vi "PV ActiveLine - Sensor On-Off (TPG361).vi"(7 "W/R":bool, 8 "Fehler (Eingang)":errorcluster, 10 "Sensor 1 Set":u8(ring) items=["No status change", "Turn gauge off", "Turn gauge on"], 11 "Referenz in":refnum<visa-resource-name>) -> (0 "Cluster (Ausgang)":errorcluster, 2 "Sensor 1 Set":u8(ring) items=["Gauge cannot be turned on/off", "Gauge turned off", "Gauge turned on"], 3 "Referenz out":refnum<visa-resource-name>)   [LabVIEW 2013, in "PV ActiveLine.lvlib"]
doc: "SEN - Turning a Gauge on/off\n\nTransmit: SEN [,a]\n\nGauge 1,\na =\n0 –> No status change\n1 –> Turn gauge off\n2 –> Turn gauge on"
uses:
  <instrlib>/PV ActiveLine/PV ActiveLine.lvlib
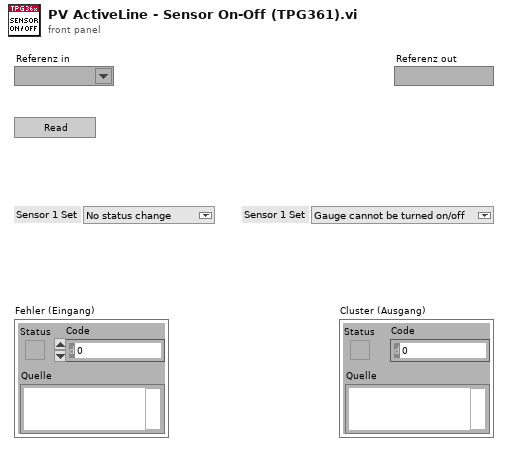
[diagram p1: front panel]
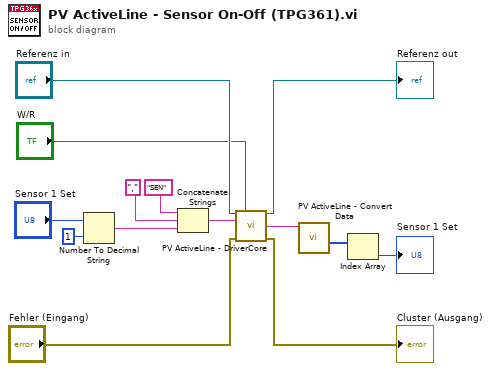
[diagram p0: block diagram]
diagram:
  n1 = Number To Decimal String(number="Sensor 1 Set", width (-)=i16 1 ("Breite (-)")) -> (decimal integer string=w4:string)
  n2 = Concatenate Strings("SEN", ",", w4) -> (w9:string)
  n3 = call <instrlib>:"PV ActiveLine - DriverCore.vi"("Referenz in"="Referenz in", "Write/Read"="W/R", "Command"=w9, "Fehler (Eingang)"="Fehler (Eingang)") -> ("Referenz out"=→"Referenz out":refnum<visa-resource-name>, "String Out"=w8:string, "Cluster (Ausgang)"=→"Cluster (Ausgang)":errorcluster)  [unwired: 9 in]
  n4 = call <instrlib>:"PV ActiveLine - Convert Data.vi"("String in"=w8) -> ("Integer Out"=w7:i32[])  [unwired: 7 in, 3 out]
  n5 = Index Array(array=w7) -> (element=→"Sensor 1 Set":i32)  [unwired: 1 in]
